vi "Lab Panel V5.20.vi"() -> ()   [LabVIEW 2013] (continued)
                            n852 = call "Save data file (stop) v3.vi"("panel id"=w1528) -> ("network file save error"=w1527:errorcluster)  [unwired: 9 in, 1 out]
                            n853 = local write "RESULT LAB04-1"(FALSE) -> ()
                            n854 = local write "data file error"(w1527) -> ()
                          }
                        }
                        n855 = Bundle(cluster=w1524, "STATUS"="STOP") -> (w1522:T4)  [unwired: 2 in]
                        n856 = local write "DISP LAB04-1"(w1522) -> ()
                      }
                    }
                  }
                  frame True {
                    n857 = local read "SIG LAB04-1"() -> (w1531:T2)
                    n858 = stacked-sequence {
                      seq-local: [w1542 _] -> [_ w1546]
                      tunnel: w1540 -> [_ w1556]
                      tunnel: w1539 -> [_ w1555]
                      tunnel: w1538 -> [_ w1554]
                      tunnel: w1537 -> [_ w1553]
                      tunnel: w1536 -> [_ w1552]
                      tunnel: [_ w1551] -> w1535
                      tunnel: w1534 -> [_ w1550]
                      tunnel: w1533 -> [_ w1549]
                      tunnel: w1532 -> [_ w1548]
                      tunnel: w1531 -> [w1541 w1547]
                      tunnel: w1530 -> [_ w1545]
                      frame #0 {
                        n859 = Unbundle(w1541) -> ("AMPS"=w1544:dbl)  [unwired: 4 out]
                        n860 = call "Check For Amps on v1.vi"("ID"="LAB04-1", "amps"=w1544) -> ("amps"=w1542:bool)  [unwired: 9 in]
                      }
                      frame #1 {
                        n861 = case shown="True" w1546 {
                          tunnel: w1556 -> [_ w1569]
                          tunnel: w1555 -> [_ w1568]
                          tunnel: w1554 -> [_ w1567]
                          tunnel: w1553 -> [_ w1566]
                          tunnel: w1552 -> [_ w1565]
                          tunnel: [errorcluster {"status"=FALSE, "code"=0, "source"=""} ("error out") w1564] -> w1551
                          tunnel: w1550 -> [_ w1563]
                          tunnel: w1549 -> [_ w1562]
                          tunnel: w1548 -> [_ w1561]
                          tunnel: w1547 -> [_ w1560]
                          tunnel: w1545 -> [_ w1559]
                          frame False {
                            w1557 = FALSE
                            n862 = local write "RUN LAB04-1"(w1557) -> ()
                            n863 = local write "run lab04-1"(w1557) -> ()
                          }
                          frame True {
                            n864 = stacked-sequence {
                              seq-local: [w1570 _ _ _ _] -> [_ w1594 _ _ _]
                              tunnel: w1569 -> [w1575 _ _ _ _]
                              tunnel: w1568 -> [w1571 _ _ _ _]
                              tunnel: w1567 -> [w1585 _ _ _ _]
                              tunnel: w1566 -> [w1578 _ _ _ _]
                              tunnel: w1565 -> [w1573 _ _ _ _]
                              tunnel: [_ w1589 _ _ _] -> w1564
                              tunnel: w1563 -> [_ _ _ w1615 _]
                              tunnel: w1562 -> [_ _ _ w1614 _]
                              tunnel: w1561 -> [_ _ _ w1613 _]
                              tunnel: w1560 -> [_ _ _ _ _]
                              tunnel: w1559 -> [_ _ _ _ w1629]
                              frame #0 {
                                w1572 = "\\"
                                n865 = local read "SET LAB04-1"() -> (w1580:T5)
                                n866 = case shown="\"CYCLE TEST\"" w1585 {
                                tunnel: ["L04-1-CHART TEST-" "L04-1-CYCLE TEST-" "L04-1-T-RISE TEST-"] -> w1581
                                frame "CHART TEST", Default {
                                }
                                frame "CYCLE TEST" {
                                }
                                frame "T-RISE TEST" {
                                }
                                }
                                n867 = Unbundle(w1580) -> ("DESCRIPTION"=w1579:string)  [unwired: 4 out]
                                n868 = Concatenate Strings(w1575, "\\", w1573, w1572, w1571, w1572) -> (w1582:string)
                                n869 = String To Path(string=w1582) -> (path=w1584:path)
                                n870 = Concatenate Strings(w1582, w1581, w1579, "-", w1578, ".tdms") -> (w1570:string)
                                n871 = Create Folder(path (use dialog)=w1584) -> (error out=w1583:errorcluster)  [unwired: 2 in, 2 out]
                                n872 = global write "Global 1.vi" "LAB04-1 FILE"(w1570) -> ()
                                n873 = call <vilib>:"Clear Errors.vi"("error in (no error)"=w1583) -> ()  [unwired: 6 in, 1 out]
                              }
                              frame #1 {
                                (unwired) FALSE
                                n874 = String To Path(string=w1594) -> (path=w1590:path)
                                n875 = TDMS Open(6:FALSE, 10:T20."create or replace" ("operation (0:open)"), 11:w1590) -> (0:w1589:errorcluster, 3:→"TDMS LAB04-1":refnum<k34>)  [unwired: 4 in]
                              }
                              frame #2 {
                                n876 = local read "SET LAB04-1"() -> (w1600:T5)
                                n877 = local read "TDMS LAB04-1"() -> (w1611:refnum<k34>)
                                n878 = Build Array("Testers Name", "Description", "Set Test Cycles", "T-Rise minutes", "T-Rise Deg C") -> (w1601:string[])
                                n879 = Unbundle(w1600) -> ("NAME"=w1599:string, "DESCRIPTION"=w1598:string, "CYCLES"=w1597:dbl, "T-RISE mins"=w1596:dbl, "T-RISE deg C"=w1595:dbl)
                                n880 = Number To Decimal String(number=w1597) -> (decimal integer string=w1610:string)  [unwired: 1 in]
                                n881 = Number To Decimal String(number=w1596) -> (decimal integer string=w1609:string)  [unwired: 1 in]
                                n882 = Number To Decimal String(number=w1595) -> (decimal integer string=w1608:string)  [unwired: 1 in]
                                n883 = Build Array(w1599, w1598, w1610, w1609, w1608) -> (w1607:string[])
                                n884 = TDMS Set Properties(5:w1607, 7:w1601, 11:w1611) -> ()  [unwired: 3 in, 4 out]
                              }
                              frame #3 {
                                n885 = local read "DISP LAB04-1"() -> (w1616:T4)
                                n886 = Concatenate Strings("LAB04-1  ", w1615) -> (w1617:string)
                                n887 = Two Button Dialog(message=w1617, 1:w1613, 2:w1614) -> (T button?=w1619:bool)
                                n888 = case shown="True" w1619 {
                                tunnel: w1616 -> [w1626 w1627]
                                tunnel: [w1626 w1627] -> w1623
                                tunnel: [w1625 w1628] -> w1622
                                tunnel: [w1624 w1628] -> w1621
                                frame False {
                                n889 = Unbundle(w1626) -> ("CYCLE"=w1625:dbl, "MINS"=w1624:dbl)  [unwired: 1 out]
                                }
                                frame True {
                                w1628 = 0.0
                                }
                                }
                                n890 = Bundle(cluster=w1623, "CYCLE"=w1622, "MINS"=w1621, "STATUS"="RUN") -> (w1612:T4)
                                n891 = local write "DISP LAB04-1"(w1612) -> ()
                              }
                              frame #4 {
                                n892 = local read "TEMP START LAB04-1"() -> (w1631:cluster{"TL":dbl, "TN":dbl})
                                n893 = Bundle(cluster=w1631, "TL"=w1629, "TN"=w1629) -> (w1630:cluster{"TL":dbl, "TN":dbl})
                                n894 = local write "TEMP START LAB04-1"(w1630) -> ()
                              }
                            }
                          }
                        }
                      }
                    }
                  }
                }
              }
              event "RUN LAB04-2": Value Change {
                n895 = event-data() -> ("NewVal"=w1636:bool)  [unwired: 1 in, 5 out]
                n896 = local write "run lab04-2"(w1636) -> ()
                n897 = case shown="True" w1636 {
                  tunnel: w1642 -> [_ w1680]
                  tunnel: w1641 -> [_ w1679]
                  tunnel: w1639 -> [w1644 w1678]
                  tunnel: w1640 -> [_ w1677]
                  tunnel: w1638 -> [_ w1676]
                  tunnel: [w1643 w1675] -> w1637
                  tunnel: w1635 -> [_ w1674]
                  tunnel: w1634 -> [_ w1673]
                  tunnel: w1633 -> [_ w1672]
                  tunnel: w1632 -> [_ w1670]
                  frame False {
                    # "stop test"
                    n898 = stacked-sequence {
                      tunnel: w1644 -> [w1653 _]
                      tunnel: [w1645 _] -> w1643
                      frame #0 {
                        n899 = local read "DISP LAB04-2"() -> (w1652:T4)
                        n900 = Unbundle(w1652) -> ("CYCLE"=w1650:dbl, "MINS"=w1651:dbl)  [unwired: 1 out]
                        n901 = case shown="\"CYCLE TEST\"" w1653 {
                          tunnel: w1651 -> [_ _ w1660]
                          tunnel: w1650 -> [w1658 w1659 _]
                          tunnel: [w1658 w1659 w1660] -> w1649
                          frame "CHART TEST", Default {
                          }
                          frame "CYCLE TEST" {
                          }
                          frame "T-RISE TEST" {
                          }
                        }
                        n902 = local read "TDMS LAB04-2"() -> (w1657:refnum<k34>)
                        n903 = Build Array("STOPPED") -> (w1654:string[])
                        n904 = Build Array(w1649) -> (w1648:dbl[])
                        n905 = TDMS Write(0:w1657, 5:"TEST RESULT", 7:w1654, 9:w1648) -> (4:w1646:refnum<k34>, 15:w1647:errorcluster)  [unwired: 2 in, 2 out]
                        n906 = TDMS Close(8:w1647, 11:w1646) -> (0:w1645:errorcluster)  [unwired: 1 out]
                      }
                      frame #1 {
                        n907 = local read "DISP LAB04-2"() -> (w1664:T4)
                        n908 = stacked-sequence {
                          tunnel: "LAB04-2" -> [w1666 w1668]
                          frame #0 {
                            n909 = call "sub vi - defrag tdms v1.vi"("panel id"=w1666) -> ("error out"=w1665:errorcluster)  [unwired: 10 in]
                            n910 = local write "data file error"(w1665) -> ()
                          }
                          frame #1 {
                            n911 = call "Save data file (stop) v3.vi"("panel id"=w1668) -> ("network file save error"=w1667:errorcluster)  [unwired: 9 in, 1 out]
                            n912 = local write "RESULT LAB04-2"(FALSE) -> ()
                            n913 = local write "data file error"(w1667) -> ()
                          }
                        }
                        n914 = Bundle(cluster=w1664, "STATUS"="STOP") -> (w1662:T4)  [unwired: 2 in]
                        n915 = local write "DISP LAB04-2"(w1662) -> ()
                      }
                    }
                  }
                  frame True {
                    n916 = local read "SIG LAB04-2"() -> (w1671:T2)
                    n917 = stacked-sequence {
                      seq-local: [w1682 _] -> [_ w1686]
                      tunnel: w1680 -> [_ w1696]
                      tunnel: w1679 -> [_ w1695]
                      tunnel: w1678 -> [_ w1694]
                      tunnel: w1677 -> [_ w1693]
                      tunnel: w1676 -> [_ w1692]
                      tunnel: [_ w1691] -> w1675
                      tunnel: w1674 -> [_ w1690]
                      tunnel: w1673 -> [_ w1689]
                      tunnel: w1672 -> [_ w1688]
                      tunnel: w1671 -> [w1681 w1687]
                      tunnel: w1670 -> [_ w1685]
                      frame #0 {
                        n918 = Unbundle(w1681) -> ("AMPS"=w1684:dbl)  [unwired: 4 out]
                        n919 = call "Check For Amps on v1.vi"("ID"="LAB04-2", "amps"=w1684) -> ("amps"=w1682:bool)  [unwired: 9 in]
                      }
                      frame #1 {
                        n920 = case shown="True" w1686 {
                          tunnel: w1696 -> [_ w1709]
                          tunnel: w1695 -> [_ w1708]
                          tunnel: w1694 -> [_ w1707]
                          tunnel: w1693 -> [_ w1706]
                          tunnel: w1692 -> [_ w1705]
                          tunnel: [errorcluster {"status"=FALSE, "code"=0, "source"=""} ("error out") w1704] -> w1691
                          tunnel: w1690 -> [_ w1703]
                          tunnel: w1689 -> [_ w1702]
                          tunnel: w1688 -> [_ w1701]
                          tunnel: w1687 -> [_ w1700]
                          tunnel: w1685 -> [_ w1699]
                          frame False {
                            w1697 = FALSE
                            n921 = local write "RUN LAB04-2"(w1697) -> ()
                            n922 = local write "run lab04-2"(w1697) -> ()
                          }
                          frame True {
                            n923 = stacked-sequence {
                              seq-local: [w1710 _ _ _ _] -> [_ w1734 _ _ _]
                              tunnel: w1709 -> [w1715 _ _ _ _]
                              tunnel: w1708 -> [w1711 _ _ _ _]
                              tunnel: w1707 -> [w1725 _ _ _ _]
                              tunnel: w1706 -> [w1718 _ _ _ _]
                              tunnel: w1705 -> [w1713 _ _ _ _]
                              tunnel: [_ w1729 _ _ _] -> w1704
                              tunnel: w1703 -> [_ _ _ w1755 _]
                              tunnel: w1702 -> [_ _ _ w1754 _]
                              tunnel: w1701 -> [_ _ _ w1753 _]
                              tunnel: w1700 -> [_ _ _ _ _]
                              tunnel: w1699 -> [_ _ _ _ w1769]
                              frame #0 {
                                w1712 = "\\"
                                n924 = local read "SET LAB04-2"() -> (w1720:T5)
                                n925 = case shown="\"CHART TEST\", Default" w1725 {
                                tunnel: ["L04-2-CHART TEST-" "L04-2-CYCLE TEST-" "L04-2-T-RISE TEST-"] -> w1721
                                frame "CHART TEST", Default {
                                }
                                frame "CYCLE TEST" {
                                }
                                frame "T-RISE TEST" {
                                }
                                }
                                n926 = Unbundle(w1720) -> ("DESCRIPTION"=w1719:string)  [unwired: 4 out]
                                n927 = Concatenate Strings(w1715, "\\", w1713, w1712, w1711, w1712) -> (w1722:string)
                                n928 = String To Path(string=w1722) -> (path=w1724:path)
                                n929 = Concatenate Strings(w1722, w1721, w1719, "-", w1718, ".tdms") -> (w1710:string)
                                n930 = Create Folder(path (use dialog)=w1724) -> (error out=w1723:errorcluster)  [unwired: 2 in, 2 out]
                                n931 = global write "Global 1.vi" "LAB04-2 FILE"(w1710) -> ()
                                n932 = call <vilib>:"Clear Errors.vi"("error in (no error)"=w1723) -> ()  [unwired: 6 in, 1 out]
                              }
                              frame #1 {
                                (unwired) FALSE
                                n933 = String To Path(string=w1734) -> (path=w1730:path)
                                n934 = TDMS Open(6:FALSE, 10:T20."create or replace" ("operation (0:open)"), 11:w1730) -> (0:w1729:errorcluster, 3:→"TDMS LAB04-2":refnum<k34>)  [unwired: 4 in]
                              }
                              frame #2 {
                                n935 = local read "SET LAB04-2"() -> (w1740:T5)
                                n936 = local read "TDMS LAB04-2"() -> (w1751:refnum<k34>)
                                n937 = Build Array("Testers Name", "Description", "Set Test Cycles", "T-Rise minutes", "T-Rise Deg C") -> (w1741:string[])
                                n938 = Unbundle(w1740) -> ("NAME"=w1739:string, "DESCRIPTION"=w1738:string, "CYCLES"=w1737:dbl, "T-RISE mins"=w1736:dbl, "T-RISE deg C"=w1735:dbl)
                                n939 = Number To Decimal String(number=w1737) -> (decimal integer string=w1750:string)  [unwired: 1 in]
                                n940 = Number To Decimal String(number=w1736) -> (decimal integer string=w1749:string)  [unwired: 1 in]
                                n941 = Number To Decimal String(number=w1735) -> (decimal integer string=w1748:string)  [unwired: 1 in]
                                n942 = Build Array(w1739, w1738, w1750, w1749, w1748) -> (w1747:string[])
                                n943 = TDMS Set Properties(5:w1747, 7:w1741, 11:w1751) -> ()  [unwired: 3 in, 4 out]
                              }
                              frame #3 {
                                n944 = local read "DISP LAB04-2"() -> (w1756:T4)
                                n945 = Concatenate Strings("LAB04-2 ", w1755) -> (w1757:string)
                                n946 = Two Button Dialog(message=w1757, 1:w1753, 2:w1754) -> (T button?=w1759:bool)
                                n947 = case shown="True" w1759 {
                                tunnel: w1756 -> [w1766 w1767]
                                tunnel: [w1766 w1767] -> w1763
                                tunnel: [w1765 w1768] -> w1762
                                tunnel: [w1764 w1768] -> w1761
                                frame False {
                                n948 = Unbundle(w1766) -> ("CYCLE"=w1765:dbl, "MINS"=w1764:dbl)  [unwired: 1 out]
                                }
                                frame True {
                                w1768 = 0.0
                                }
                                }
                                n949 = Bundle(cluster=w1763, "CYCLE"=w1762, "MINS"=w1761, "STATUS"="RUN") -> (w1752:T4)
                                n950 = local write "DISP LAB04-2"(w1752) -> ()
                              }
                              frame #4 {
                                n951 = local read "TEMP START LAB04-2"() -> (w1771:cluster{"TL":dbl, "TN":dbl})
                                n952 = Bundle(cluster=w1771, "TL"=w1769, "TN"=w1769) -> (w1770:cluster{"TL":dbl, "TN":dbl})
                                n953 = local write "TEMP START LAB04-2"(w1770) -> ()
                              }
                            }
                          }
                        }
                      }
                    }
                  }
                }
              }
              event "RUN LAB05-1": Value Change {
                n954 = event-data() -> ("NewVal"=w1776:bool)  [unwired: 1 in, 5 out]
                n955 = local write "run lab05-1"(w1776) -> ()
                n956 = case shown="True" w1776 {
                  tunnel: w1782 -> [_ w1820]
                  tunnel: w1781 -> [_ w1819]
                  tunnel: w1779 -> [w1784 w1818]
                  tunnel: w1780 -> [_ w1817]
                  tunnel: w1778 -> [_ w1816]
                  tunnel: [w1783 w1815] -> w1777
                  tunnel: w1775 -> [_ w1814]
                  tunnel: w1774 -> [_ w1813]
                  tunnel: w1773 -> [_ w1812]
                  tunnel: w1772 -> [_ w1810]
                  frame False {
                    # "stop test"
                    n957 = stacked-sequence {
                      tunnel: w1784 -> [w1793 _]
                      tunnel: [w1785 _] -> w1783
                      frame #0 {
                        n958 = local read "DISP LAB05-1"() -> (w1792:T4)
                        n959 = Unbundle(w1792) -> ("CYCLE"=w1790:dbl, "MINS"=w1791:dbl)  [unwired: 1 out]
                        n960 = case shown="\"CYCLE TEST\"" w1793 {
                          tunnel: w1791 -> [_ _ w1800]
                          tunnel: w1790 -> [w1798 w1799 _]
                          tunnel: [w1798 w1799 w1800] -> w1789
                          frame "CHART TEST", Default {
                          }
                          frame "CYCLE TEST" {
                          }
                          frame "T-RISE TEST" {
                          }
                        }
                        n961 = local read "TDMS LAB05-1"() -> (w1797:refnum<k34>)
                        n962 = Build Array("STOPPED") -> (w1794:string[])
                        n963 = Build Array(w1789) -> (w1788:dbl[])
                        n964 = TDMS Write(0:w1797, 5:"TEST RESULT", 7:w1794, 9:w1788) -> (4:w1786:refnum<k34>, 15:w1787:errorcluster)  [unwired: 2 in, 2 out]
                        n965 = TDMS Close(8:w1787, 11:w1786) -> (0:w1785:errorcluster)  [unwired: 1 out]
                      }
                      frame #1 {
                        n966 = local read "DISP LAB05-1"() -> (w1804:T4)
                        n967 = stacked-sequence {
                          tunnel: "LAB05-1" -> [w1806 w1808]
                          frame #0 {
                            n968 = call "sub vi - defrag tdms v1.vi"("panel id"=w1806) -> ("error out"=w1805:errorcluster)  [unwired: 10 in]
                            n969 = local write "data file error"(w1805) -> ()
                          }
                          frame #1 {
                            n970 = call "Save data file (stop) v3.vi"("panel id"=w1808) -> ("network file save error"=w1807:errorcluster)  [unwired: 9 in, 1 out]
                            n971 = local write "RESULT LAB05-1"(FALSE) -> ()
                            n972 = local write "data file error"(w1807) -> ()
                          }
                        }
                        n973 = Bundle(cluster=w1804, "STATUS"="STOP") -> (w1802:T4)  [unwired: 2 in]
                        n974 = local write "DISP LAB05-1"(w1802) -> ()
                      }
                    }
                  }
                  frame True {
                    n975 = local read "SIG LAB05-1"() -> (w1811:T2)
                    n976 = stacked-sequence {
                      seq-local: [w1822 _] -> [_ w1826]
                      tunnel: w1820 -> [_ w1836]
                      tunnel: w1819 -> [_ w1835]
                      tunnel: w1818 -> [_ w1834]
                      tunnel: w1817 -> [_ w1833]
                      tunnel: w1816 -> [_ w1832]
                      tunnel: [_ w1831] -> w1815
                      tunnel: w1814 -> [_ w1830]
                      tunnel: w1813 -> [_ w1829]
                      tunnel: w1812 -> [_ w1828]
                      tunnel: w1811 -> [w1821 w1827]
                      tunnel: w1810 -> [_ w1825]
                      frame #0 {
                        n977 = Unbundle(w1821) -> ("AMPS"=w1824:dbl)  [unwired: 4 out]
                        n978 = call "Check For Amps on v1.vi"("ID"="LAB05-1", "amps"=w1824) -> ("amps"=w1822:bool)  [unwired: 9 in]
                      }
                      frame #1 {
                        n979 = case shown="True" w1826 {
                          tunnel: w1836 -> [_ w1849]
                          tunnel: w1835 -> [_ w1848]
                          tunnel: w1834 -> [_ w1847]
                          tunnel: w1833 -> [_ w1846]
                          tunnel: w1832 -> [_ w1845]
                          tunnel: [errorcluster {"status"=FALSE, "code"=0, "source"=""} ("error out") w1844] -> w1831
                          tunnel: w1830 -> [_ w1843]
                          tunnel: w1829 -> [_ w1842]
                          tunnel: w1828 -> [_ w1841]
                          tunnel: w1827 -> [_ w1840]
                          tunnel: w1825 -> [_ w1839]
                          frame False {
                            w1837 = FALSE
                            n980 = local write "RUN LAB05-1"(w1837) -> ()
                            n981 = local write "run lab05-1"(w1837) -> ()
                          }
                          frame True {
                            n982 = stacked-sequence {
                              seq-local: [w1850 _ _ _ _] -> [_ w1874 _ _ _]
                              tunnel: w1849 -> [w1855 _ _ _ _]
                              tunnel: w1848 -> [w1851 _ _ _ _]
                              tunnel: w1847 -> [w1865 _ _ _ _]
                              tunnel: w1846 -> [w1858 _ _ _ _]
                              tunnel: w1845 -> [w1853 _ _ _ _]
                              tunnel: [_ w1869 _ _ _] -> w1844
                              tunnel: w1843 -> [_ _ _ w1894 _]
                              tunnel: w1842 -> [_ _ _ w1893 _]
                              tunnel: w1841 -> [_ _ _ w1892 _]
                              tunnel: w1840 -> [_ _ _ _ _]
                              tunnel: w1839 -> [_ _ _ _ w1909]
                              frame #0 {
                                w1852 = "\\"
                                n983 = local read "SET LAB05-1"() -> (w1860:T5)
                                n984 = case shown="\"CYCLE TEST\"" w1865 {
                                tunnel: ["L05-1-CHART TEST-" "L05-1-CYCLE TEST-" "L05-1-T-RISE TEST-"] -> w1861
                                frame "CHART TEST", Default {
                                }
                                frame "CYCLE TEST" {
                                }
                                frame "T-RISE TEST" {
                                }
                                }
                                n985 = Unbundle(w1860) -> ("DESCRIPTION"=w1859:string)  [unwired: 4 out]
                                n986 = Concatenate Strings(w1855, "\\", w1853, w1852, w1851, w1852) -> (w1862:string)
                                n987 = String To Path(string=w1862) -> (path=w1864:path)
                                n988 = Concatenate Strings(w1862, w1861, w1859, "-", w1858, ".tdms") -> (w1850:string)
                                n989 = Create Folder(path (use dialog)=w1864) -> (error out=w1863:errorcluster)  [unwired: 2 in, 2 out]
                                n990 = global write "Global 1.vi" "LAB05-1 FILE"(w1850) -> ()
                                n991 = call <vilib>:"Clear Errors.vi"("error in (no error)"=w1863) -> ()  [unwired: 6 in, 1 out]
                              }
                              frame #1 {
                                (unwired) FALSE
                                n992 = String To Path(string=w1874) -> (path=w1870:path)
                                n993 = TDMS Open(6:FALSE, 10:T20."create or replace" ("operation (0:open)"), 11:w1870) -> (0:w1869:errorcluster, 3:→"TDMS LAB05-1":refnum<k34>)  [unwired: 4 in]
                              }
                              frame #2 {
                                n994 = local read "SET LAB05-1"() -> (w1880:T5)
                                n995 = local read "TDMS LAB05-1"() -> (w1891:refnum<k34>)
                                n996 = Build Array("Testers Name", "Description", "Set Test Cycles", "T-Rise minutes", "T-Rise Deg C") -> (w1881:string[])
                                n997 = Unbundle(w1880) -> ("NAME"=w1879:string, "DESCRIPTION"=w1878:string, "CYCLES"=w1877:dbl, "T-RISE mins"=w1876:dbl, "T-RISE deg C"=w1875:dbl)
                                n998 = Number To Decimal String(number=w1877) -> (decimal integer string=w1890:string)  [unwired: 1 in]
                                n999 = Number To Decimal String(number=w1876) -> (decimal integer string=w1889:string)  [unwired: 1 in]
                                n1000 = Number To Decimal String(number=w1875) -> (decimal integer string=w1888:string)  [unwired: 1 in]
                                n1001 = Build Array(w1879, w1878, w1890, w1889, w1888) -> (w1887:string[])
                                n1002 = TDMS Set Properties(5:w1887, 7:w1881, 11:w1891) -> ()  [unwired: 3 in, 4 out]
                              }
                              frame #3 {
                                n1003 = local read "DISP LAB05-1"() -> (w1896:T4)
                                n1004 = Concatenate Strings("LAB05-1  ", w1894) -> (w1897:string)
                                n1005 = Two Button Dialog(message=w1897, 1:w1892, 2:w1893) -> (T button?=w1899:bool)
                                n1006 = case shown="True" w1899 {
                                tunnel: w1896 -> [w1906 w1907]
                                tunnel: [w1906 w1907] -> w1903
                                tunnel: [w1905 w1908] -> w1902
                                tunnel: [w1904 w1908] -> w1901
                                frame False {
                                n1007 = Unbundle(w1906) -> ("CYCLE"=w1905:dbl, "MINS"=w1904:dbl)  [unwired: 1 out]
                                }
                                frame True {
                                w1908 = 0.0
                                }
                                }
                                n1008 = Bundle(cluster=w1903, "CYCLE"=w1902, "MINS"=w1901, "STATUS"="RUN") -> (w1895:T4)
                                n1009 = local write "DISP LAB05-1"(w1895) -> ()
                              }
                              frame #4 {
                                n1010 = local read "TEMP START LAB05-1"() -> (w1911:cluster{"TL":dbl, "TN":dbl})
                                n1011 = Bundle(cluster=w1911, "TL"=w1909, "TN"=w1909) -> (w1910:cluster{"TL":dbl, "TN":dbl})
                                n1012 = local write "TEMP START LAB05-1"(w1910) -> ()
                              }
                            }
                          }
                        }
                      }
                    }
                  }
                }
              }
              event "RUN LAB05-2": Value Change {
                n1013 = event-data() -> ("NewVal"=w1917:bool)  [unwired: 1 in, 5 out]
                n1014 = local read "SIG LAB05-2"() -> (w1913:T2)
                n1015 = case shown="True" w1917 {
                  tunnel: w1923 -> [_ w1961]
                  tunnel: w1922 -> [_ w1960]
                  tunnel: w1920 -> [w1925 w1959]
                  tunnel: w1921 -> [_ w1958]
                  tunnel: w1919 -> [_ w1957]
                  tunnel: [w1924 w1956] -> w1918
                  tunnel: w1916 -> [_ w1955]
                  tunnel: w1915 -> [_ w1954]
                  tunnel: w1914 -> [_ w1953]
                  tunnel: w1913 -> [_ w1952]
                  tunnel: w1912 -> [_ w1951]
                  frame False {
                    # "stop test"
                    n1016 = stacked-sequence {
                      tunnel: w1925 -> [w1934 _]
                      tunnel: [w1926 _] -> w1924
                      frame #0 {
                        n1017 = local read "DISP LAB05-2"() -> (w1933:T4)
                        n1018 = Unbundle(w1933) -> ("CYCLE"=w1931:dbl, "MINS"=w1932:dbl)  [unwired: 1 out]
                        n1019 = case shown="\"CYCLE TEST\"" w1934 {
                          tunnel: w1932 -> [_ _ w1941]
                          tunnel: w1931 -> [w1939 w1940 _]
                          tunnel: [w1939 w1940 w1941] -> w1930
                          frame "CHART TEST", Default {
                          }
                          frame "CYCLE TEST" {
                          }
                          frame "T-RISE TEST" {
                          }
                        }
                        n1020 = local read "TDMS LAB05-2"() -> (w1938:refnum<k34>)
                        n1021 = Build Array("STOPPED") -> (w1935:string[])
                        n1022 = Build Array(w1930) -> (w1929:dbl[])
                        n1023 = TDMS Write(0:w1938, 5:"TEST RESULT", 7:w1935, 9:w1929) -> (4:w1927:refnum<k34>, 15:w1928:errorcluster)  [unwired: 2 in, 2 out]
                        n1024 = TDMS Close(8:w1928, 11:w1927) -> (0:w1926:errorcluster)  [unwired: 1 out]
                      }
                      frame #1 {
                        n1025 = local read "DISP LAB05-2"() -> (w1945:T4)
                        n1026 = stacked-sequence {
                          tunnel: "LAB05-2" -> [w1947 w1949]
                          frame #0 {
                            n1027 = call "sub vi - defrag tdms v1.vi"("panel id"=w1947) -> ("error out"=w1946:errorcluster)  [unwired: 10 in]
                            n1028 = local write "data file error"(w1946) -> ()
                          }
                          frame #1 {
                            n1029 = local write "RESULT LAB05-2"(FALSE) -> ()
                            n1030 = call "Save data file (stop) v3.vi"("panel id"=w1949) -> ("network file save error"=w1948:errorcluster)  [unwired: 9 in, 1 out]
                            n1031 = local write "data file error"(w1948) -> ()
                          }
                        }
                        n1032 = Bundle(cluster=w1945, "STATUS"="STOP") -> (w1943:T4)  [unwired: 2 in]
                        n1033 = local write "DISP LAB05-2"(w1943) -> ()
                      }
                    }
                  }
                  frame True {
                    n1034 = stacked-sequence {
                      seq-local: [w1963 _] -> [_ w1967]
                      tunnel: w1961 -> [_ w1977]
                      tunnel: w1960 -> [_ w1976]
                      tunnel: w1959 -> [_ w1975]
                      tunnel: w1958 -> [_ w1974]
                      tunnel: w1957 -> [_ w1973]
                      tunnel: [_ w1972] -> w1956
                      tunnel: w1955 -> [_ w1971]
                      tunnel: w1954 -> [_ w1970]
                      tunnel: w1953 -> [_ w1969]
                      tunnel: w1952 -> [w1962 w1968]
                      tunnel: w1951 -> [_ w1966]
                      frame #0 {
                        n1035 = Unbundle(w1962) -> ("AMPS"=w1965:dbl)  [unwired: 4 out]
                        n1036 = call "Check For Amps on v1.vi"("ID"="LAB05-2", "amps"=w1965) -> ("amps"=w1963:bool)  [unwired: 9 in]
                      }
                      frame #1 {
                        n1037 = case shown="True" w1967 {
                          tunnel: w1977 -> [_ w1990]
                          tunnel: w1976 -> [_ w1989]
                          tunnel: w1975 -> [_ w1988]
                          tunnel: w1974 -> [_ w1987]
                          tunnel: w1973 -> [_ w1986]
                          tunnel: [errorcluster {"status"=FALSE, "code"=0, "source"=""} ("error out") w1985] -> w1972
                          tunnel: w1971 -> [_ w1984]
                          tunnel: w1970 -> [_ w1983]
                          tunnel: w1969 -> [_ w1982]
                          tunnel: w1968 -> [_ w1981]
                          tunnel: w1966 -> [_ w1980]
                          frame False {
                            w1978 = FALSE
                            n1038 = local write "RUN LAB05-2"(w1978) -> ()
                            n1039 = local write "run lab05-2"(w1978) -> ()
                          }
                          frame True {
                            n1040 = stacked-sequence {
                              seq-local: [w1991 _ _ _ _] -> [_ w2015 _ _ _]
                              tunnel: w1990 -> [w1996 _ _ _ _]
                              tunnel: w1989 -> [w1992 _ _ _ _]
                              tunnel: w1988 -> [w2006 _ _ _ _]
                              tunnel: w1987 -> [w1999 _ _ _ _]
                              tunnel: w1986 -> [w1994 _ _ _ _]
                              tunnel: [_ w2010 _ _ _] -> w1985
                              tunnel: w1984 -> [_ _ _ w2035 _]
                              tunnel: w1983 -> [_ _ _ w2034 _]
                              tunnel: w1982 -> [_ _ _ w2033 _]
                              tunnel: w1981 -> [_ _ _ _ _]
                              tunnel: w1980 -> [_ _ _ _ w2050]
                              frame #0 {
                                w1993 = "\\"
                                n1041 = local read "SET LAB05-2"() -> (w2001:T5)
                                n1042 = case shown="\"CYCLE TEST\"" w2006 {
                                tunnel: ["L05-2-CHART TEST-" "L05-2-CYCLE TEST-" "L05-2-T-RISE TEST-"] -> w2002
                                frame "CHART TEST", Default {
                                }
                                frame "CYCLE TEST" {
                                }
                                frame "T-RISE TEST" {
                                }
                                }
                                n1043 = Unbundle(w2001) -> ("DESCRIPTION"=w2000:string)  [unwired: 4 out]
                                n1044 = Concatenate Strings(w1996, "\\", w1994, w1993, w1992, w1993) -> (w2003:string)
                                n1045 = String To Path(string=w2003) -> (path=w2005:path)
                                n1046 = Concatenate Strings(w2003, w2002, w2000, "-", w1999, ".tdms") -> (w1991:string)
                                n1047 = Create Folder(path (use dialog)=w2005) -> (error out=w2004:errorcluster)  [unwired: 2 in, 2 out]
                                n1048 = global write "Global 1.vi" "LAB05-2 FILE"(w1991) -> ()
                                n1049 = call <vilib>:"Clear Errors.vi"("error in (no error)"=w2004) -> ()  [unwired: 6 in, 1 out]
                              }
                              frame #1 {
                                (unwired) FALSE
                                n1050 = String To Path(string=w2015) -> (path=w2011:path)
                                n1051 = TDMS Open(6:FALSE, 10:T20."create or replace" ("operation (0:open)"), 11:w2011) -> (0:w2010:errorcluster, 3:→"TDMS LAB05-2":refnum<k34>)  [unwired: 4 in]
                              }
                              frame #2 {
                                n1052 = local read "SET LAB05-2"() -> (w2021:T5)
                                n1053 = local read "TDMS LAB05-2"() -> (w2032:refnum<k34>)
                                n1054 = Build Array("Testers Name", "Description", "Set Test Cycles", "T-Rise minutes", "T-Rise Deg C") -> (w2022:string[])
                                n1055 = Unbundle(w2021) -> ("NAME"=w2020:string, "DESCRIPTION"=w2019:string, "CYCLES"=w2018:dbl, "T-RISE mins"=w2017:dbl, "T-RISE deg C"=w2016:dbl)
                                n1056 = Number To Decimal String(number=w2018) -> (decimal integer string=w2031:string)  [unwired: 1 in]
                                n1057 = Number To Decimal String(number=w2017) -> (decimal integer string=w2030:string)  [unwired: 1 in]
                                n1058 = Number To Decimal String(number=w2016) -> (decimal integer string=w2029:string)  [unwired: 1 in]
                                n1059 = Build Array(w2020, w2019, w2031, w2030, w2029) -> (w2028:string[])
                                n1060 = TDMS Set Properties(5:w2028, 7:w2022, 11:w2032) -> ()  [unwired: 3 in, 4 out]
                              }
                              frame #3 {
                                n1061 = local read "DISP LAB05-2"() -> (w2037:T4)
                                n1062 = Concatenate Strings("LAB05-2  ", w2035) -> (w2038:string)
                                n1063 = Two Button Dialog(message=w2038, 1:w2033, 2:w2034) -> (T button?=w2040:bool)
                                n1064 = case shown="True" w2040 {
                                tunnel: w2037 -> [w2047 w2048]
                                tunnel: [w2047 w2048] -> w2044
                                tunnel: [w2046 w2049] -> w2043
                                tunnel: [w2045 w2049] -> w2042
                                frame False {
                                n1065 = Unbundle(w2047) -> ("CYCLE"=w2046:dbl, "MINS"=w2045:dbl)  [unwired: 1 out]
                                }
                                frame True {
                                w2049 = 0.0
                                }
                                }
                                n1066 = Bundle(cluster=w2044, "CYCLE"=w2043, "MINS"=w2042, "STATUS"="RUN") -> (w2036:T4)
                                n1067 = local write "DISP LAB05-2"(w2036) -> ()
                              }
                              frame #4 {
                                n1068 = local read "TEMP START LAB05-2"() -> (w2052:cluster{"TL":dbl, "TN":dbl})
                                n1069 = Bundle(cluster=w2052, "TL"=w2050, "TN"=w2050) -> (w2051:cluster{"TL":dbl, "TN":dbl})
                                n1070 = local write "TEMP START LAB05-2"(w2051) -> ()
                              }
                            }
                          }
                        }
                      }
                    }
                  }
                }
                n1071 = local write "run lab05-2"(w1917) -> ()
              }
            }
            n1072 = local write "data file error"(w621) -> ()
          }
          frame #4 {
            # "check if test cycles reached for cycle tests, if so then test pass"
            n1073 = stacked-sequence {
              tunnel: w2072 -> [_ _ _ _ _ _ _ _ _ _]
              tunnel: w2071 -> [_ _ _ _ _ _ _ _ _ _]
              tunnel: w2070 -> [_ _ _ _ _ _ _ _ _ _]
              tunnel: w2069 -> [_ _ _ _ _ _ _ _ _ _]
              tunnel: w2068 -> [_ _ _ _ _ _ _ _ _ _]
              tunnel: w2067 -> [_ _ _ _ _ _ _ _ _ _]
              tunnel: w2066 -> [_ _ _ _ _ _ _ _ _ _]
              tunnel: w2065 -> [_ _ _ _ _ _ _ _ _ _]
              tunnel: w2064 -> [_ _ _ _ _ _ _ _ _ _]
              tunnel: w2063 -> [_ _ _ _ _ _ _ _ _ _]
              tunnel: w2062 -> [w2078 _ _ _ _ _ _ _ _ _]
              tunnel: w2061 -> [_ w2113 _ _ _ _ _ _ _ _]
              tunnel: w2060 -> [_ _ w2153 _ _ _ _ _ _ _]
              tunnel: w2059 -> [_ _ _ w2193 _ _ _ _ _ _]
              tunnel: w2058 -> [_ _ _ _ w2233 _ _ _ _ _]
              tunnel: w2057 -> [_ _ _ _ _ w2273 _ _ _ _]
              tunnel: w2056 -> [_ _ _ _ _ _ w2313 _ _ _]
              tunnel: w2055 -> [_ _ _ _ _ _ _ w2353 _ _]
              tunnel: w2054 -> [_ _ _ _ _ _ _ _ w2393 _]
              tunnel: w2053 -> [_ _ _ _ _ _ _ _ _ w2433]
              frame #0 {
                # "LAB01-1"
                n1074 = Less?(x=w2078, y=2) -> (x < y?=w2076:bool)
                n1075 = local read "DISP LAB01-1"() -> (w2079:T4)
                n1076 = Unbundle(w2079) -> ("STATUS"=w2073:string)  [unwired: 2 out]
                n1077 = Equal?(x=w2073, y="RUN") -> (x = y?=w2075:bool)
                n1078 = And(x=w2075, y=w2076) -> (x .and. y?=w2074:bool)
                n1079 = case shown="True" w2074 {
                  tunnel: w2079 -> [_ w2084]
                  tunnel: w2078 -> [_ w2088]
                  frame False {
                  }
                  frame True {
                    n1080 = local read "SET LAB01-1"() -> (w2090:T5)
                    n1081 = local read "TDMS LAB01-1"() -> (w2083:refnum<k34>)
                    n1082 = Unbundle(w2090) -> ("CYCLES"=w2081:dbl, "T-RISE mins"=w2087:dbl)  [unwired: 3 out]
                    n1083 = case shown="\"CYCLE TEST\"" w2088 {
                      tunnel: w2087 -> [_ _ w2097]
                      tunnel: [w2092 w2094 w2097] -> w2086
                      tunnel: w2081 -> [w2092 w2094 _]
                      tunnel: ["CHART PASS" "CYCLE PASS" "T-RISE PASS"] -> w2085
                      frame "CHART TEST", Default {
                      }
                      frame "CYCLE TEST" {
                      }
                      frame "T-RISE TEST" {
                      }
                    }
                    n1084 = Unbundle(w2084) -> ("CYCLE"=w2089:dbl)  [unwired: 2 out]
                    n1085 = Increment(x=w2081) -> (x+1=w2082:dbl)
                    n1086 = Greater Or Equal?(x=w2089, y=w2082) -> (x >= y?=w2091:bool)
                    n1087 = case shown="True" w2091 {
                      tunnel: w2086 -> [w2101 _]
                      tunnel: w2085 -> [w2100 _]
                      tunnel: w2084 -> [w2099 _]
                      tunnel: w2083 -> [w2098 _]
                      frame True {
                        n1088 = stacked-sequence {
                          tunnel: w2101 -> [w2105 _]
                          tunnel: w2100 -> [w2103 w2109]
                          tunnel: w2099 -> [_ w2112]
                          tunnel: w2098 -> [w2102 _]
                          frame #0 {
                            n1089 = Build Array(w2103) -> (w2106:string[])
                            n1090 = Build Array(w2105) -> (w2104:dbl[])
                            n1091 = TDMS Write(0:w2102, 5:"TEST PASS", 7:w2106, 9:w2104) -> (15:w2108:errorcluster)  [unwired: 2 in, 3 out]
                            n1092 = local write "data file error"(w2108) -> ()
                          }
                          frame #1 {
                            n1093 = Bundle(cluster=w2112, "STATUS"=w2109) -> (w2110:T4)  [unwired: 2 in]
                            n1094 = local write "RESULT LAB01-1"(TRUE) -> ()
                            n1095 = local write "DISP LAB01-1"(w2110) -> ()
                          }
                        }
                      }
                      frame False {
                      }
                    }
                  }
                }
              }
              frame #1 {
                # "LAB01-2"
                n1096 = Less?(x=w2113, y=2) -> (x < y?=w2116:bool)
                n1097 = local read "DISP LAB01-2"() -> (w2118:T4)
                n1098 = Unbundle(w2118) -> ("STATUS"=w2119:string)  [unwired: 2 out]
                n1099 = Equal?(x=w2119, y="RUN") -> (x = y?=w2115:bool)
                n1100 = And(x=w2115, y=w2116) -> (x .and. y?=w2114:bool)
                n1101 = case shown="True" w2114 {
                  tunnel: w2118 -> [_ w2124]
                  tunnel: w2113 -> [_ w2128]
                  frame False {
                  }
                  frame True {
                    n1102 = local read "SET LAB01-2"() -> (w2130:T5)
                    n1103 = local read "TDMS LAB01-2"() -> (w2123:refnum<k34>)
                    n1104 = Unbundle(w2130) -> ("CYCLES"=w2121:dbl, "T-RISE mins"=w2127:dbl)  [unwired: 3 out]
                    n1105 = case shown="\"T-RISE TEST\"" w2128 {
                      tunnel: w2127 -> [_ _ w2137]
                      tunnel: [w2132 w2134 w2137] -> w2126
                      tunnel: w2121 -> [w2132 w2134 _]
                      tunnel: ["CHART PASS" "CYCLE PASS" "T-RISE PASS"] -> w2125
                      frame "CHART TEST", Default {
                      }
                      frame "CYCLE TEST" {
                      }
                      frame "T-RISE TEST" {
                      }
                    }
                    n1106 = Unbundle(w2124) -> ("CYCLE"=w2129:dbl)  [unwired: 2 out]
                    n1107 = Increment(x=w2121) -> (x+1=w2122:dbl)
                    n1108 = Greater Or Equal?(x=w2129, y=w2122) -> (x >= y?=w2131:bool)
                    n1109 = case shown="True" w2131 {
                      tunnel: w2126 -> [w2141 _]
                      tunnel: w2125 -> [w2140 _]
                      tunnel: w2124 -> [w2139 _]
                      tunnel: w2123 -> [w2138 _]
                      frame True {
                        n1110 = stacked-sequence {
                          tunnel: w2141 -> [w2145 _]
                          tunnel: w2140 -> [w2143 w2149]
                          tunnel: w2139 -> [_ w2152]
                          tunnel: w2138 -> [w2142 _]
                          frame #0 {
                            n1111 = Build Array(w2143) -> (w2146:string[])
                            n1112 = Build Array(w2145) -> (w2144:dbl[])
                            n1113 = TDMS Write(0:w2142, 5:"TEST PASS", 7:w2146, 9:w2144) -> (15:w2148:errorcluster)  [unwired: 2 in, 3 out]
                            n1114 = local write "data file error"(w2148) -> ()
                          }
                          frame #1 {
                            n1115 = Bundle(cluster=w2152, "STATUS"=w2149) -> (w2150:T4)  [unwired: 2 in]
                            n1116 = local write "RESULT LAB01-2"(TRUE) -> ()
                            n1117 = local write "DISP LAB01-2"(w2150) -> ()
                          }
                        }
                      }
                      frame False {
                      }
                    }
                  }
                }
              }
              frame #2 {
                # "LAB02-1"
                n1118 = Less?(x=w2153, y=2) -> (x < y?=w2156:bool)
                n1119 = local read "DISP LAB02-1"() -> (w2158:T4)
                n1120 = Unbundle(w2158) -> ("STATUS"=w2159:string)  [unwired: 2 out]
                n1121 = Equal?(x=w2159, y="RUN") -> (x = y?=w2155:bool)
                n1122 = And(x=w2155, y=w2156) -> (x .and. y?=w2154:bool)
                n1123 = case shown="True" w2154 {
                  tunnel: w2158 -> [_ w2164]
                  tunnel: w2153 -> [_ w2168]
                  frame False {
                  }
                  frame True {
                    n1124 = local read "SET LAB02-1"() -> (w2170:T5)
                    n1125 = local read "TDMS LAB02-1"() -> (w2163:refnum<k34>)
                    n1126 = Unbundle(w2164) -> ("CYCLE"=w2169:dbl)  [unwired: 2 out]
                    n1127 = Unbundle(w2170) -> ("CYCLES"=w2161:dbl, "T-RISE mins"=w2167:dbl)  [unwired: 3 out]
                    n1128 = case shown="\"T-RISE TEST\"" w2168 {
                      tunnel: w2167 -> [_ _ w2177]
